vi "Asana_Post_Comment.vi"() -> ()   [LabVIEW 2016]
uses:
  <vilib>/httpClient/POSTBuffer.vi
  <vilib>/httpClient/LabVIEWHTTPClient.lvlib
panel:
  out "Status":string
  out "HTTP Returned Body":string
  out "HTTP Returned Headers":string
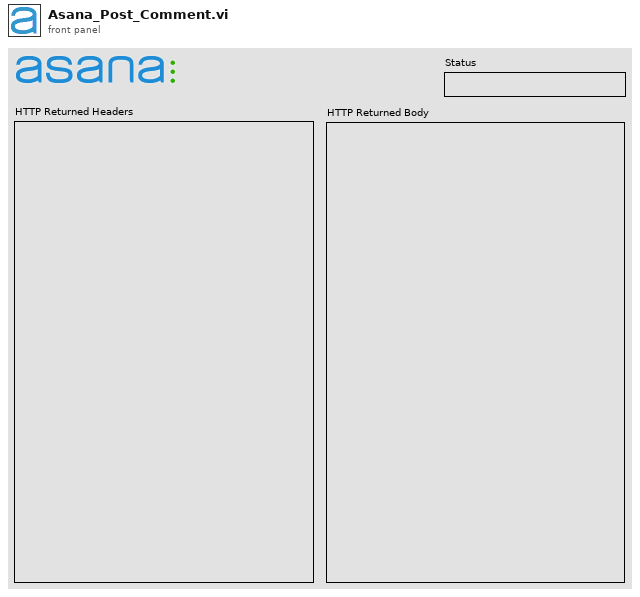
[diagram p1: front panel]
types:
  T1 = typedef "LabVIEWHTTPClient.lvlib/ClientHandle.ctl" = refnum<k1>
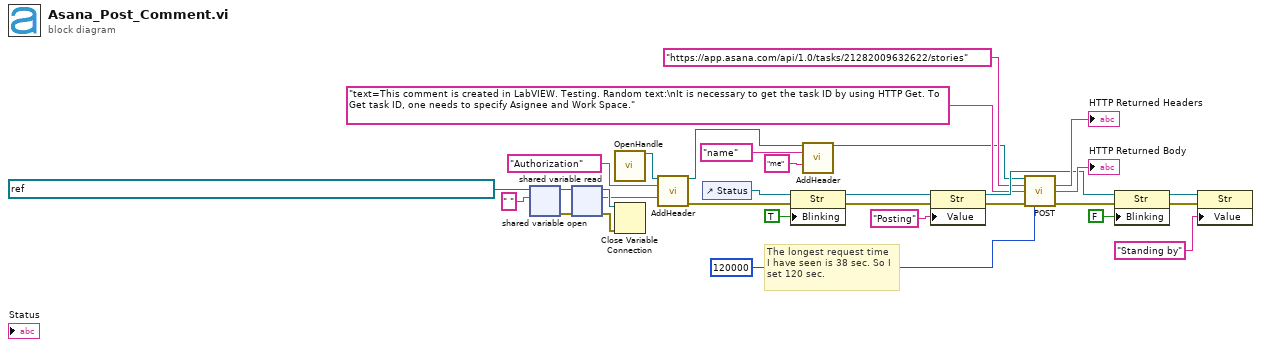
[diagram p0: block diagram]
diagram:
  # "The longest request time\nI have seen is 38 sec. So I\nset 120 sec."
  n1 = shared-variable-open(refnum<k21> "ni.var.psp://housesoftheholy/OneNote API HTTP/Asana Access Token 15669051163913" ("shared variable refnum in"), " " ("string")) -> (w25:refnum<k21>, w24:errorcluster)  [unwired: 2 in]
  n2 = shared-variable-read(w25, w24) -> (w22:refnum<k21>, w23:errorcluster, w21:string)  [unwired: 1 out]
  n3 = call <vilib>:"OpenHandle.vi"() -> ("client handle out"=w29:T1)  [unwired: 14 in, 1 out]
  n4 = Close Variable Connection(8:w23, 11:w22) -> ()  [unwired: 1 out]
  n5 = call <vilib>:"AddHeader.vi"("client handle"=w29, "header"="Authorization", "value"=w21) -> ("client handle out"=w2:T1, "error out"=w6:errorcluster)  [unwired: 11 in]
  n6 = control-ref of="Status"() -> (w14:refnum<vi>)
  n7 = property on="Property Node" class="Str"(reference=w14, error in=w6, "Blinking"=TRUE) -> (reference out=w13:refnum<vi>, error out=w12:errorcluster)
  n8 = call <vilib>:"AddHeader.vi"("client handle"=w2, "header"="name", "value"="me") -> ("client handle out"=w1:T1)  [unwired: 11 in, 1 out]
  n9 = property on="Property Node" class="Str"(reference=w13, error in=w12, "Value"="Posting" ("Status")) -> (reference out=w10:refnum<vi>, error out=w11:errorcluster)
  n10 = call-poly <vilib>:"POST.vi"("client handle"=w1, "url"="https://app.asana.com/api/1.0/tasks/21282009632622/stories", "buffer"="text=This comment is created in LabVIEW. Testing. Random text:\nIt is necessary to get the task ID by using HTTP Get. To Get task ID, one needs to specify Asignee and Work Space.", "error in (no error)"=w11, "timeout (10000)"=120000) -> ("headers"=→"HTTP Returned Headers":string, "body"=→"HTTP Returned Body":string, "error out"=w9:errorcluster)  [unwired: 7 in, 1 out]
  n11 = property on="Property Node" class="Str"(reference=w10, error in=w9, "Blinking"=FALSE ("Visible")) -> (reference out=w8:refnum<vi>, error out=w15:errorcluster)
  n12 = property on="Property Node" class="Str"(reference=w8, error in=w15, "Value"="Standing by" ("Status")) -> ()  [unwired: 2 out]
